vi "fifo_test.vi"() -> ()   [LabVIEW 2017]
uses:
  <vilib>/rvi/Emulation/niFpgaGetClockAttributes.vi
  <vilib>/rvi/Emulation/niFpgaSctlEmulationGetInTimedLoop.vi
  <vilib>/rvi/Emulation/niFpgaEmulationReportErrorSimple.vi
  <vilib>/rvi/interface/RandomDataEmulation/niFpgaRandomDataHandleErrors.vi
  <vilib>/rvi/Emulation/niFpgaCriticalErrorInLSC.vi
  <vilib>/rvi/DataTransferAndStorage/Container/XNode/niFpgaContainer.xnode
  <vilib>/rvi/interface/RandomDataEmulation/nirviRandomDataFpgaReadWriteTemplate.vi
  <vilib>/rvi/Analysis/measure/butterworth/XNode/niFpgaButterworthFilter.xnode
panel:
  out "Waveform Chart":sgl(graph)
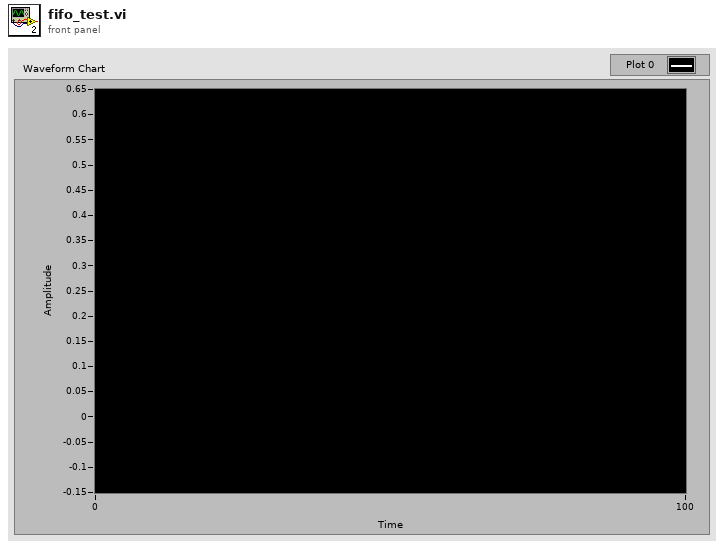
[diagram p1: front panel]
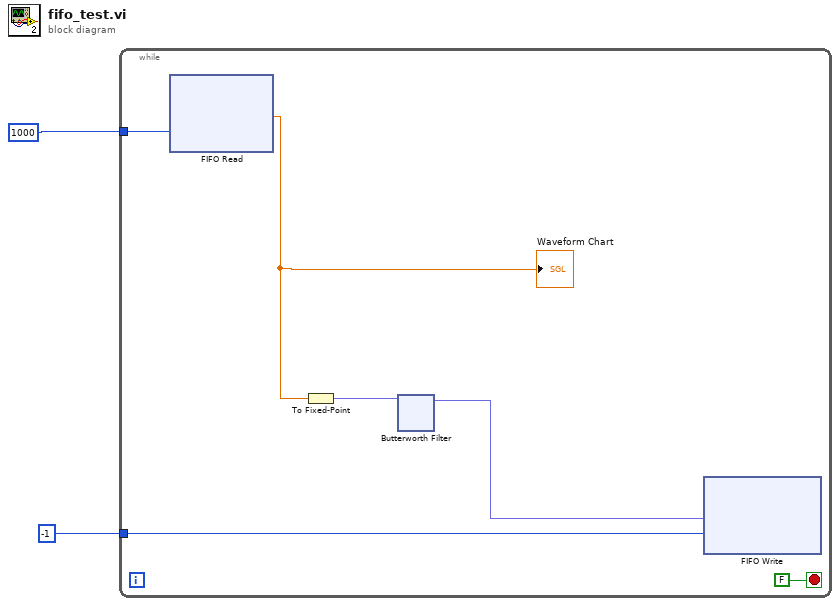
[diagram p0: block diagram]
diagram:
  n1 = while {
    tunnel: i16 1000 -> [w7]
    tunnel: i16 -1 -> [w6]
    stop <- FALSE stop-if-true
    n2 = xnode "FIFO Read"("Timeout"=w7) -> ("Element"=w4:sgl)  [unwired: 1 in, 2 out]
    "Waveform Chart" <- w4
    n3 = To Fixed-Point(number=w4) -> (fixed-point=w5:fxp<+/-,32,16>)  [unwired: 1 in]
    n4 = xnode "Butterworth Filter"("input data"=w5) -> ("output data"=w3:fxp<+/-,36,20>)  [unwired: 2 in]
    n5 = xnode "FIFO Write"("Element"=w3, "Timeout"=w6) -> ()  [unwired: 1 in, 2 out]
  }
